vi "plotTest.vi"(10 "Current Temp":dbl, 11 "Room Temperure (K)":refnum<vi>) -> (2 "Current Temperature":dbl, 3 "Temperature (K)":dbl(graph))   [LabVIEW 2013]
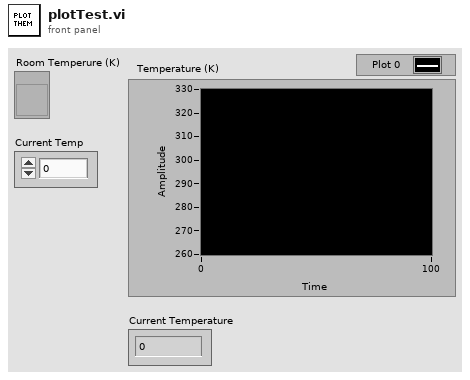
[diagram p1: front panel]
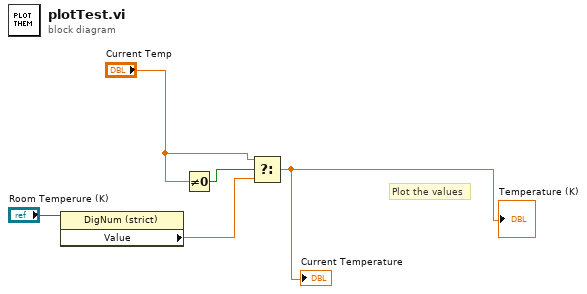
[diagram p0: block diagram]
diagram:
  # "Plot the values"
  n1 = property on="Property Node" class="DigNum (strict)"(reference="Room Temperure (K)") -> ("Value"=w4:dbl)  [unwired: 1 in, 2 out]
  n2 = Not Equal To 0?(x="Current Temp") -> (x != 0?=w2:bool)
  n3 = Select(t="Current Temp", s=w2, f=w4) -> (s? t:f=→"Temperature (K)" →"Current Temperature":dbl)
